vi "InGaAs_error_detected.vi"() -> ()   [LabVIEW 2020]
panel:
  out "Returned Array":i32[](array[numeric])
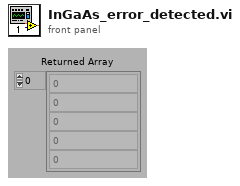
[diagram p1: front panel]
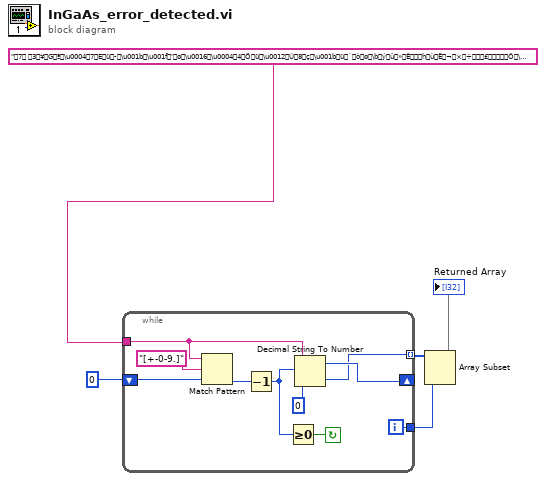
[diagram p0: block diagram]
diagram:
  n1 = while {
    tunnel: "7 3¥Gª\u00047Eü-\u001b\u001f'ø\u0016\u00044Öü\u0012Ú8ç\u001bü´òø\býû»ÊhùË¬×÷£Ô\u0011Qã" -> [w7]
    tunnel: [w8] -> w3
    tunnel: [w9] -> w4 mode=indexing
    shift-left: 0 -> [w14]
    shift-right: [w10] -> _
    i -> [w8]
    stop <- w6 continue-if-true
    n2 = Match Pattern(string=w7, regular expression="[+-0-9.]", offset (0)=w14) -> (offset past match=w13:i32)  [unwired: 3 out]
    n3 = Decrement(x=w13) -> (x-1=w11:i32)
    n4 = Greater Or Equal To 0?(x=w11) -> (x >= 0?=w6:bool)
    n5 = Decimal String To Number(string=w7, offset=w11, default (0L)=0) -> (offset past number=w10:i32, number=w9:i32)
  }
  n6 = Array Subset(array=w4, length=w3) -> (→"Returned Array":i32[])  [unwired: 1 in]
